vi "SxmPlane.vi"() -> ()   [LabVIEW 2021]
uses:
  <vilib>/Analysis/6fits.llb/Curve Fitting Criteria.ctl
  <vilib>/Analysis/baseanly.llb/Mean (DBL).vi
  <userlib>/Nanonis Prog Interface V5/Nanonis Prog Interface.lvlib
  <vilib>/Analysis/NI_AALBase.lvlib
  <vilib>/Analysis/NI_AALPro.lvlib
panel:
  out "x-axis(3pt)":dbl=0.8796796142820119
  out "y-axis (3pt)":dbl=-1.842025740138959
  in  "quardrantsize":i32=2
  in  "Datafile (1=last)":i32=1
  out "x*y":dbl[](array[numeric])=[-0.0, 0.0, 5.267119811214001e-24]
  in  "method":T1 items=["Least Square", "Least Absolute Residual", "Bisquare"]
  in  "index":i32
  out "Saved file path":path=path "D:/STM Data/082016/160824_13-54-30_SPM001.sxm"
  out "Pixelated 2":picture
  out "y-axis Deg":dbl=-1.849984543458349
  out "x-axis Deg":dbl=0.9660828184327803
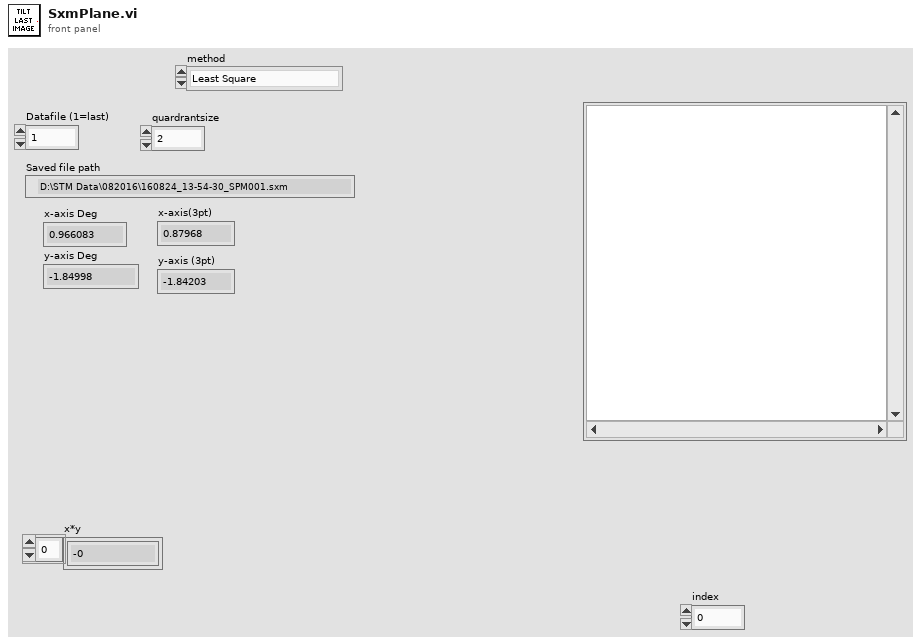
[diagram p1: front panel]
types:
  T1 = typedef "NI_AALPro.lvlib/Curve Fitting Criteria.ctl" = u16
  T2 = cluster{"center X":sgl, "center Y":sgl, "angle":sgl, "width":sgl, "height":sgl, "# pixels":i32, "# lines":i32}
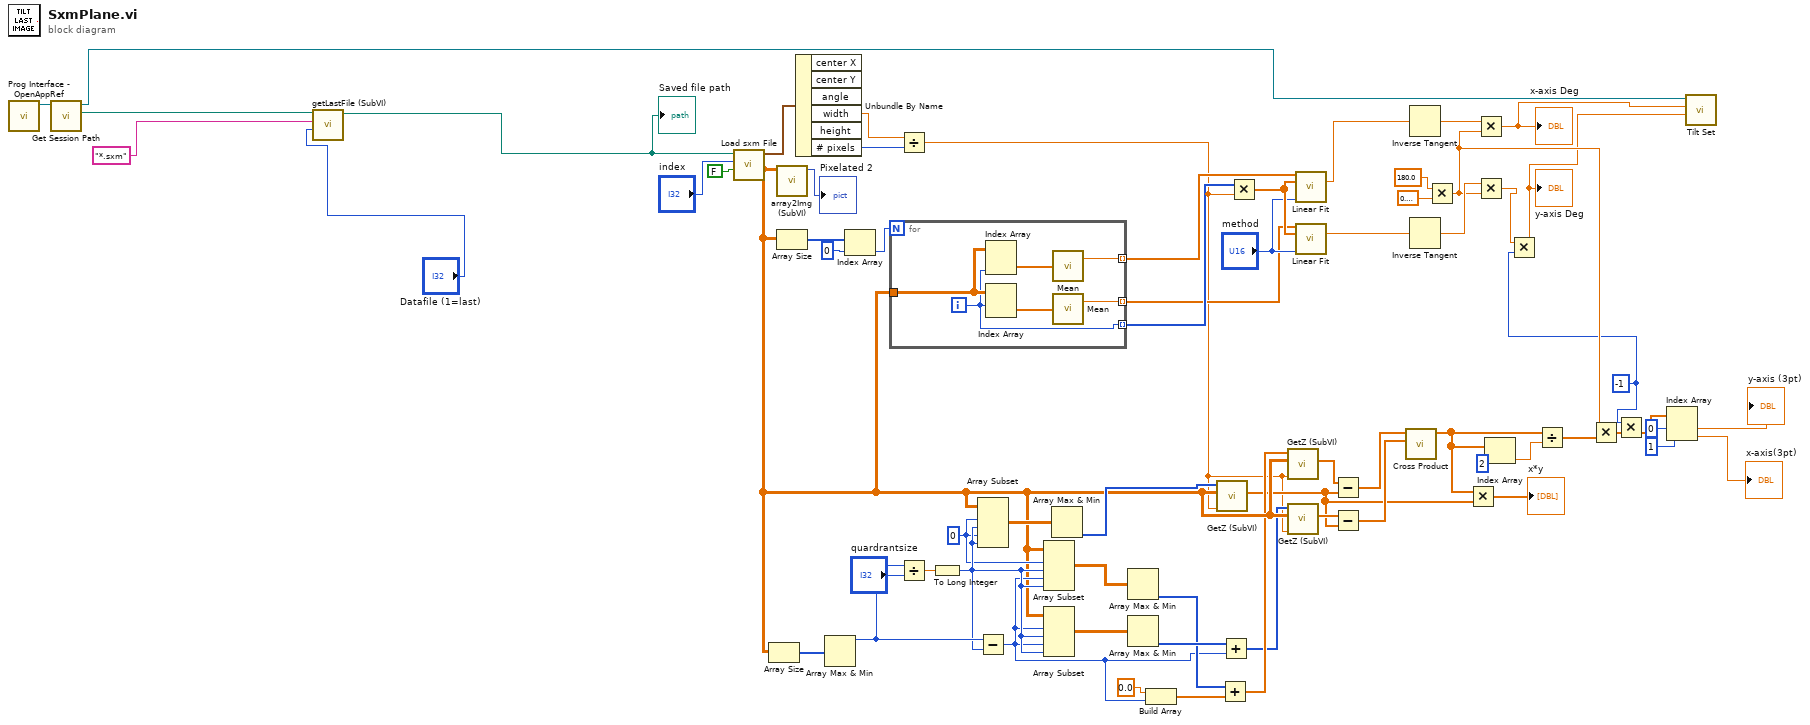
[diagram p0: block diagram]
diagram:
  w4 = -1 ("index")
  w35 = 0 ("index")
  n1 = call <userlib>:"Prog Interface - OpenAppRef.vi"() -> ("Application reference"=w57:refnum<vi>)  [unwired: 6 in, 1 out]
  n2 = call <userlib>:"Get Session Path.vi"("Application ref in"=w57) -> ("Session path"=w56:path, "Application ref out"=w3:refnum<vi>)  [unwired: 8 in, 1 out]
  n3 = call "getLastFile (SubVI).vi"("Datafile (1=last)"="Datafile (1=last)", "pattern"="*.sxm", "Session path"=w56) -> ("path out"=w55:path)  [unwired: 8 in]
  "Saved file path" <- w55
  n4 = call <userlib>:"Load sxm File.vi"("Scan direction"=FALSE, "Read channel"="index", "Scan data file"=w55) -> ("Data"=w28:sgl[][], "Scanfield"=w52:T2)  [unwired: 3 in, 4 out]
  n5 = Array Size(array=w28) -> (size(s)=w42:i32[])
  n6 = call "array2Img (SubVI).vi"("Rxy"=w28) -> ("new picture"=→"Pixelated 2":picture)  [unwired: 10 in]
  n7 = Array Size(array=w28) -> (size(s)=w65:i32[])
  n8 = Unbundle By Name(w52) -> ("width"=w51:sgl, "# pixels"=w50:i32)  [unwired: 4 out]
  n9 = Array Max & Min(array=w42) -> (max value=w40:i32)  [unwired: 3 out]
  n10 = Index Array(array=w65, index=0) -> (element=w62:i32)
  n11 = for {
    N: w62 -> [_]
    tunnel: w28 -> [w72]
    tunnel: [w67] -> w63 mode=indexing
    tunnel: [w69] -> w44 mode=indexing
    tunnel: [w68] -> w43 mode=indexing
    i -> [w67]
    n12 = Index Array(array=w72, index (col)=w67) -> (element=w70:sgl[])  [unwired: 1 in]
    n13 = Index Array(array=w72, index (row)=w67) -> (element=w71:sgl[])  [unwired: 1 in]
    n14 = call-poly <vilib>:"Mean.vi"("X"=w70) -> ("mean"=w68:dbl)  [unwired: 1 out]
    n15 = call-poly <vilib>:"Mean.vi"("X"=w71) -> ("mean"=w69:dbl)  [unwired: 1 out]
  }
  n16 = Divide(x=w51, y=w50) -> (x/y=w13:sgl)
  n17 = Divide(x=w40, y="quardrantsize") -> (x/y=w41:dbl)
  n18 = To Long Integer(number=w41) -> (32bit integer=w36:i32)
  n19 = Array Subset(array=w28, index (row)=w35, length (row)=w36, index (col)=w35, length (col)=w36) -> (w39:sgl[][])
  n20 = Subtract(x=w40, y=w36) -> (x-y=w31:i32)
  n21 = Array Subset(array=w28, index (row)=w35, length (row)=w36, index (col)=w31, length (col)=w36) -> (w34:sgl[][])
  n22 = Array Subset(array=w28, index (row)=w31, length (row)=w36, index (col)=w31, length (col)=w36) -> (w38:sgl[][])
  n23 = Array Max & Min(array=w39) -> (min index (indices)=w29:i32[])  [unwired: 3 out]
  n24 = Array Max & Min(array=w34) -> (min index (indices)=w33:i32[])  [unwired: 3 out]
  n25 = Array Max & Min(array=w38) -> (min index (indices)=w37:i32[])  [unwired: 3 out]
  n26 = Build Array(0.0 ("element"), w31) -> (w30:dbl[])
  n27 = call "GetZ (SubVI).vi"("calibration"=w13, "Data"=w28, "Array"=w29) -> ("appended array"=w21:sgl[])  [unwired: 5 in, 3 out]
  n28 = Add(x=w33, y=w30) -> (x+y=w27:dbl[])
  n29 = Add(x=w37, y=w31) -> (x+y=w26:i32[])
  n30 = Multiply(x=w63, y=w13) -> (x*y=w53:sgl[])
  n31 = call "GetZ (SubVI).vi"("calibration"=w13, "Data"=w28, "Array"=w27) -> ("appended array"=w25:sgl[])  [unwired: 5 in, 3 out]
  n32 = call "GetZ (SubVI).vi"("calibration"=w13, "Data"=w28, "Array"=w26) -> ("appended array"=w24:sgl[])  [unwired: 5 in, 3 out]
  n33 = call <vilib>:"Linear Fit.vi"("Y"=w43, "X"=w53, "method"="method") -> ("slope"=w61:dbl)  [unwired: 8 in, 4 out]
  n34 = call <vilib>:"Linear Fit.vi"("Y"=w44, "X"=w53, "method"="method") -> ("slope"=w60:dbl)  [unwired: 8 in, 4 out]
  n35 = Subtract(x=w25, y=w21) -> (x-y=w23:sgl[])
  n36 = Subtract(x=w24, y=w21) -> (x-y=w22:sgl[])
  n37 = call <vilib>:"Cross Product.vi"("B Vector"=w22, "A Vector"=w23) -> ("Cross Product"=w18:dbl[])  [unwired: 8 in, 1 out]
  n38 = Inverse Tangent(1:w61) -> (0:w46:dbl)
  n39 = Inverse Tangent(1:w60) -> (0:w47:dbl)
  n40 = Multiply(x=180.0, y=0.3183098861837907) -> (x*y=w14:dbl)
  n41 = Multiply(x=w18, y=w21) -> (x*y=→"x*y":dbl[])
  n42 = Multiply(x=w46, y=w14) -> (x*y=w2:dbl)
  "x-axis Deg" <- w2
  n43 = Multiply(x=w47, y=w14) -> (x*y=w5:dbl)
  n44 = Index Array(array=w18, index=2) -> (element=w15:dbl)
  n45 = Multiply(x=w5, y=w4) -> (x*y=w1:dbl)
  "y-axis Deg" <- w1
  n46 = Divide(x=w18, y=w15) -> (x/y=w16:dbl[])
  n47 = Multiply(x=w14, y=w16) -> (x*y=w11:dbl[])
  n48 = Multiply(x=w4, y=w11) -> (x*y=w6:dbl[])
  n49 = Index Array(array=w6, index #1=0 ("index"), index #2=1 ("index")) -> (element #1=→"y-axis (3pt)":dbl, element #2=→"x-axis(3pt)":dbl)
  n50 = call <userlib>:"Tilt Set.vi"("Tilt Y (deg)"=w1, "Tilt X (deg)"=w2, "Application ref in"=w3) -> ()  [unwired: 7 in, 2 out]
